vi "emi_Window Store Position in Ini.vi"(2 "Section(VI Name)":string, 5 "VI Refnum(This VI)":refnum<vi>, 9 "error in (no error)":errorcluster) -> (6 "VI Refnum":refnum<vi>, 10 "error out":errorcluster)   [LabVIEW 2011]
doc: "Store the window position, and splitters in ini file.\n\nOn error: Do nothing"
uses:
  0 - General/App/emi_Application Folder.vi
  <vilib>/Utility/libraryn.llb/Check if File or Folder Exists.vi
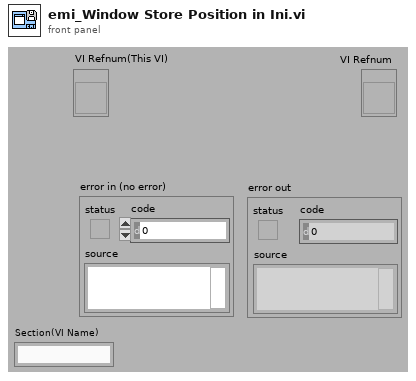
[diagram p1: front panel]
types:
  T1 = enum32{"Invalid", "Standard", "Closed", "Hidden", "Minimized", "Maximized"}
  T2 = typedef "LVRectTypeDef.ctl" = cluster{"left":i16, "top":i16, "right":i16, "bottom":i16}
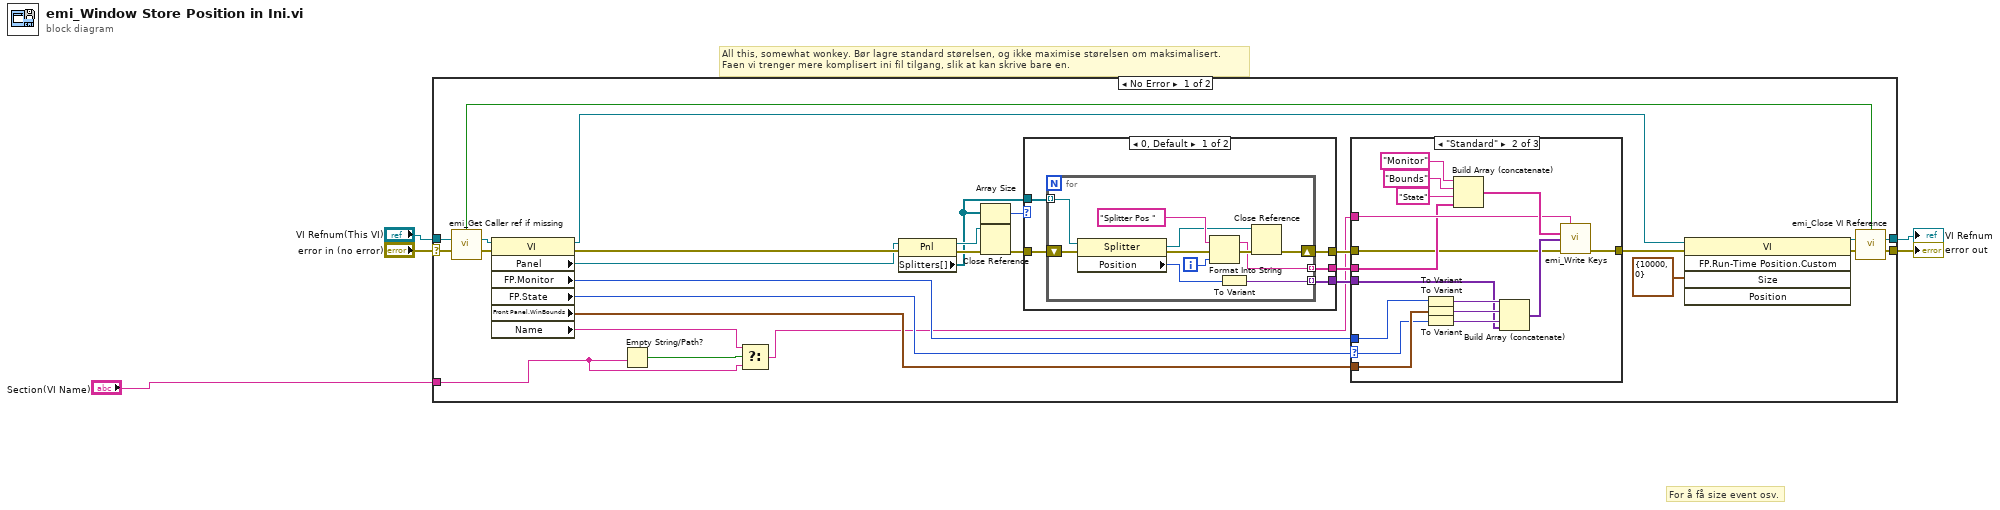
[diagram p0: block diagram]
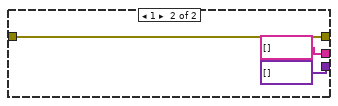
[diagram p2: hidden frame]
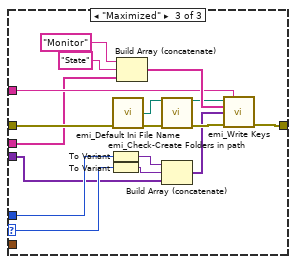
[diagram p4: hidden frame]
diagram:
  # "For å få size event osv."
  # "All this, somewhat wonkey. Bør lagre standard størelsen, og ikke maximise størelsen om maksimalisert.\nFaen vi trenger mere komplisert ini fil tilgang, slik at kan skrive bare en."
  n1 = case shown="No Error" "error in (no error)" {
    selector: "error in (no error)" -> [w26 w88]
    tunnel: "VI Refnum(This VI)" -> [w30 w89]
    tunnel: [w29 w88] -> w4
    tunnel: [w28 w89] -> w3
    tunnel: "Section(VI Name)" -> [w8 _]
    frame No Error {
      n2 = call "emi_Get Caller ref if missing.vi"("VI Refnum(Calling VI)"=w30, "error in (no error)"=w26) -> ("Ref Generated"=w27:bool, "VI Refnum Out"=w32:refnum<vi>, "error out"=w31:errorcluster)  [unwired: 11 in]
      n3 = property class="VI"(reference=w32, error in=w31) -> (reference out=w12:refnum<vi>, error out=w23:errorcluster, "Panel"=w22:refnum<vi>, "FP.Monitor"=w25:u16, "FP.State"=w33:T1, "Front Panel.WinBounds"=w34:T2, "Name"=w7:string)
      n4 = Empty String/Path?(string/path=w8) -> (empty?=w9:bool)
      n5 = Select(t=w7, s=w9, f=w8) -> (s? t:f=w6:string)
      n6 = property class="Pnl"(reference=w22, error in=w23) -> (reference out=w24:refnum<vi>, error out=w21:errorcluster, "Splitters[]"=w17:refnum<vi>[])
      n7 = Array Size(array=w17) -> (size(s)=w20:i32)
      n8 = Close Reference(reference=w24, error in (no error)=w21) -> (error out=w19:errorcluster)
      n9 = case shown="0, Default" w20 {
        tunnel: w19 -> [w39 w53]
        tunnel: [w38 w53] -> w18
        tunnel: w17 -> [w37 _]
        tunnel: [w36 string[] []] -> w16
        tunnel: [w35 variant[] []] -> w15
        frame 0, Default {
          n10 = for {
            tunnel: w37 -> [w44] mode=indexing
            tunnel: [w43] -> w36 mode=indexing
            tunnel: [w40] -> w35 mode=indexing
            shift-right: [w45] -> w38
            shift-left: w39 -> [w46]
            i -> [w42]
            n11 = property class="Splitter"(reference=w44, error in=w46) -> (reference out=w47:refnum<vi>, error out=w49:errorcluster, "Position"=w41:i32)
            n12 = Format Into String(initial string="Splitter Pos ", error in=w49, w42) -> (resulting string=w43:string, error out=w50:errorcluster)  [unwired: 1 in]
            n13 = To Variant(anything=w41) -> (Variant=w40:variant)
            n14 = Close Reference(reference=w47, error in (no error)=w50) -> (error out=w45:errorcluster)
          }
        }
        frame 1 {
        }
      }
      n15 = case shown="\"Standard\"" w33 {
        selector: w33 -> [_ w59 w76]
        tunnel: w18 -> [w54 w55 w85]
        tunnel: [w54 w70 w84] -> w14
        tunnel: w25 -> [_ w61 w77]
        tunnel: w34 -> [_ w60 _]
        tunnel: w6 -> [_ w58 w75]
        tunnel: w16 -> [_ w56 w71]
        tunnel: w15 -> [_ w57 w72]
        frame "Invalid", Default {
        }
        frame "Standard" {
          n16 = To Variant(anything=w61) -> (Variant=w65:variant)
          n17 = To Variant(anything=w60) -> (Variant=w64:variant)
          n18 = To Variant(anything=w59) -> (Variant=w63:variant)
          n19 = Build Array (concatenate)("Monitor" ("Name"), "Bounds" ("Name"), "State" ("element"), w56) -> (w66:string[])
          n20 = Build Array (concatenate)(w65, w64, w63, w57) -> (w62:variant[])
          n21 = call "emi_Write Keys.vi"("Section"=w58, "Key Names"=w66, "Values"=w62, "error in (no error)"=w55) -> ("error out"=w70:errorcluster)  [unwired: 10 in, 1 out]
        }
        frame "Maximized" {
          n22 = To Variant(anything=w77) -> (Variant=w80:variant)
          n23 = To Variant(anything=w76) -> (Variant=w79:variant)
          n24 = call "emi_Default Ini File Name.vi"("error in (no error)"=w85) -> ("Path"=w74:path, "error out"=w87:errorcluster)  [unwired: 13 in]
          n25 = Build Array (concatenate)("Monitor" ("Name"), "State" ("element"), w71) -> (w81:string[])
          n26 = call "emi_Check-Create Folders in path.vi"("Path including file"=w74, "error in (no error)"=w87) -> ("Path out"=w73:path, "error out"=w86:errorcluster)  [unwired: 11 in, 1 out]
          n27 = Build Array (concatenate)(w80, w79, w72) -> (w78:variant[])
          n28 = call "emi_Write Keys.vi"("Ini Path(..app../config.ini)"=w73, "Section"=w75, "Key Names"=w81, "Values"=w78, "error in (no error)"=w86) -> ("error out"=w84:errorcluster)  [unwired: 9 in, 1 out]
        }
      }
      n29 = invoke class="VI" method="FP.Run-Time Position.Custom"(reference=w12, error in=w14, "Size"=cluster{"Top":i16, "Left":i16} {"Top"=10000, "Left"=0} ("Position")) -> (reference out=w11:refnum<vi>, error out=w13:errorcluster)  [unwired: 2 in, 3 out]
      n30 = call "emi_Close VI Reference.vi"("Close ref?(T)"=w27, "VI Refnum"=w11, "error in (no error)"=w13) -> ("VI Refnum Out"=w28:refnum<vi>, "error out"=w29:errorcluster)  [unwired: 11 in]
    }
    frame Error {
    }
  }
  "error out" <- w4
  "VI Refnum" <- w3
